vi "PH_Waveplate-GUI_6P.PC_Settings.vi"(0 "i ref in":refnum<vi>, 5 "error in":errorcluster) -> (14 "i ref out":refnum<vi>, 19 "error out":errorcluster)   [LabVIEW 2014, in "PH_Waveplate-GUI_6P.lvlib"]
uses:
  PH_Waveplate-GUI_6P.lvlib
  PH_AxisGUI_BaseClass/PH_AxisGUI_BaseClass.lvlib
  PH_Common/PH_Common.lvlib
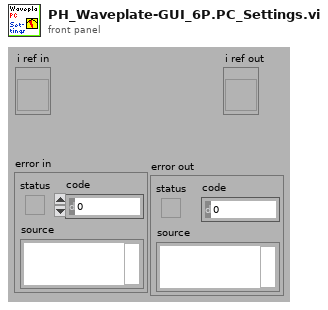
[diagram p1: front panel]
types:
  T1 = typedef "PH_AxisGUI_BaseClass.lvlib/PH_AxisGUI_BaseClass.i attribute.ctl" = cluster{"Axes":T2[]}
  T2 = typedef "PH_AxisGUI_BaseClass.lvlib/PH_AxisGUI_BaseClass.Axis Attributes.ctl" = cluster{"Axis GUI Refs":T3, "Address":T4, "Name":string, "Label \"Back\"":string, "Labell \"Forth\"":string, "Moving?":bool}
  T3 = typedef "PH_AxisGUI_BaseClass.lvlib/PH_AxisGUI_BaseClass.Axis GUI Refs.ctl" = cluster{"Back":refnum<vi>, "Forth":refnum<vi>, "Status":refnum<vi>, "Target":refnum<vi>, "Address":refnum<vi>, "Status Bar":refnum<vi>, "Settings":refnum<vi>, "Activity":refnum<vi>, "Clear Error":refnum<vi>}
  T4 = typedef "PH_Stepmotor_BaseClass.lvlib/PH_Stepmotor_BaseClass.Axis Address.ctl" = cluster{"Instance":string, "Motor Nr":i32}
  T5 = typedef "PH_Waveplate-GUI_6P.lvlib/PH_Waveplate-GUI_6P.i attribute.ctl" = cluster{"GUI Refs":cluster{"Meter":refnum<vi>, "Extend Limits":refnum<vi>, "Type":refnum<vi>, "Target":refnum<vi>}, "Extend Waveplate Limit":bool, "Type":T6, "Limit":dbl}
  T6 = typedef "PH_Waveplate-GUI_6P.lvlib/PH_Waveplate-GUI_6P.Type.ctl" = u16
  T7 = typedef "PH_Stepmotor_BaseClass.lvlib/PH_Stepmotor_BaseClass.Axis Settings.ctl" = cluster{"Sign change":bool, "Width":dbl, "Calibration":dbl, "Unit":string, "Motor Type":T8, "Unit Width":string, "Unit CF":string}
  T8 = typedef "PH_Stepmotor_BaseClass.lvlib/PH_Stepmotor_BaseClass.Motor Type.ctl" = enum16{"Unspecific", "OWIS 49.120.2633", "OWIS 49.060.1033", "OWIS 43.040.2558", "Diamond Motion 2200 series", "OWIS 49.120.266B.MV6", "Calorimeter", "Linear Stage 1", "MICOS VT-80", "MICOS VT-80 S", "Standa Rotstage nt0.95A", "PUF RA 320.200", "PUF RA 800.200", "PUF RA 800.400", "PUF RA 400.50", "1324.nn.800.50", "1324.n9c.800.50", "1324.nn.320.200", "1324.nn.400.200", "1324.nn.800.200", "1324.nn.400.50", "1324.8c9c.800.50", "1324.8c9c.400.200"}
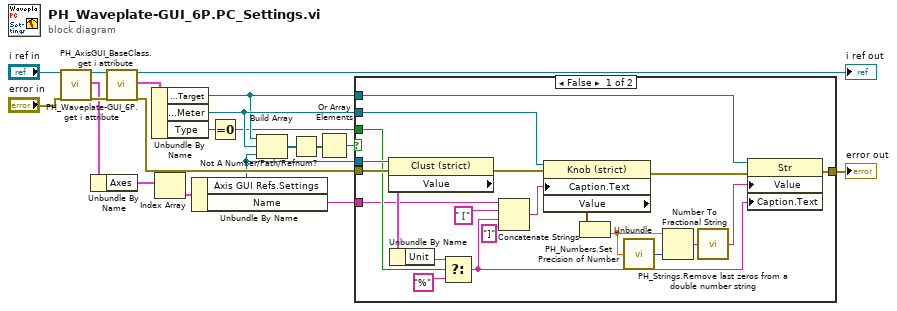
[diagram p0: block diagram]
diagram:
  n1 = call "PH_AxisGUI_BaseClass.get i attribute.vi"("i ref in"="i ref in", "error in (no error)"="error in") -> ("i ref out"=w8:refnum<vi>, "i attribute"=w7:T1, "error out"=w10:errorcluster)  [unwired: 15 in]
  n2 = Unbundle By Name(w7) -> ("Axes"=w6:T2[])
  n3 = call "PH_Waveplate-GUI_6P.get i attribute.vi"("i ref in"=w8, "error in (no error)"=w10) -> ("i ref out"=→"i ref out":refnum<vi>, "i attribute"=w18:T5, "error out"=w12:errorcluster)  [unwired: 15 in]
  n4 = Unbundle By Name(w18) -> ("GUI Refs.Target"=w11:refnum<vi>, "GUI Refs.Meter"=w14:refnum<vi>, "Type"=w3:T6)
  n5 = Index Array(array=w6) -> (element=w5:T2)  [unwired: 1 in]
  n6 = Unbundle By Name(w5) -> ("Axis GUI Refs.Settings"=w4:refnum<vi>, "Name"=w1:string)
  n7 = Equal To 0?(x=w3) -> (x = 0?=w2:bool)
  n8 = Build Array(w11, w14, w4) -> (w15:refnum<vi>[])
  n9 = Not A Number/Path/Refnum?(number/path/refnum=w15) -> (NaN/Path/Refnum?=w16:bool[])
  n10 = Or Array Elements(Boolean array=w16) -> (logical OR=w17:bool)
  n11 = case shown="False" w17 {
    tunnel: w12 -> [w36 w42]
    tunnel: [w41 w42] -> w20
    tunnel: w11 -> [w38 _]
    tunnel: w14 -> [w39 _]
    tunnel: w4 -> [w34 _]
    tunnel: w2 -> [w31 _]
    tunnel: w1 -> [w25 _]
    frame False {
      n12 = property class="Clust (strict)"(reference=w34, error in=w36) -> (error out=w35:errorcluster, "Value"=w33:T7)  [unwired: 1 out]
      n13 = Unbundle By Name(w33) -> ("Unit"=w30:string)
      n14 = Select(t=w30, s=w31, f="%" ("Unit")) -> (s? t:f=w26:string)
      n15 = Concatenate Strings(w25, " [" ("string"), w26, "]" ("string")) -> (w24:string)
      n16 = property class="Knob (strict)"(reference=w39, error in=w35, "Caption.Text"=w24) -> (error out=w37:errorcluster, "Value"=w29:cluster{dbl, dbl})  [unwired: 1 out]
      n17 = Unbundle(w29) -> (w23:dbl)  [unwired: 1 out]
      n18 = call "PH_Numbers.Set Precision of Number.vi"("Number"=w23) -> ("Precision"=w22:i16)
      n19 = Number To Fractional String(number=w23, precision (6)=w22) -> (F-format string=w40:string)  [unwired: 2 in]
      n20 = call "PH_Strings.Remove last zeros from a double number string.vi"("String in"=w40) -> ("String out"=w21:string)
      n21 = property class="Str"(reference=w38, error in=w37, "Value"=w21, "Caption.Text"=w26) -> (error out=w41:errorcluster)  [unwired: 1 out]
    }
    frame True {
    }
  }
  "error out" <- w20
